vi "Stop.vi"(8 "error in (no error)":errorcluster, 11 "TELEDINE_LECROY in":refnum<class "TELEDINE_LECROY.lvclass">) -> (0 "error out":errorcluster, 3 "TELEDINE_LECROY out":refnum<class "TELEDINE_LECROY.lvclass">)   [LabVIEW 2018, in "TELEDINE_LECROY.lvclass"]
uses:
  TELEDINE_LECROY.lvclass
  C:/Users/Sergey Denisov/Documents/REPS/TRANCON/Classes/GeneralFunctionality/GeneralFunctionality.lvclass
  C:/Users/Sergey Denisov/Documents/REPS/TRANCON/Classes/Oscilloscope/Oscilloscope.lvclass
  GeneralFunctionality/GeneralFunctionality.lvclass/GeneralFunctionality.ctl
  Oscilloscope.lvclass/Oscilloscope.ctl
  LeCroy Wave Series/LeCroy Wave Series.lvlib
  Oscilloscope.lvclass
  GeneralFunctionality/GeneralFunctionality.lvclass
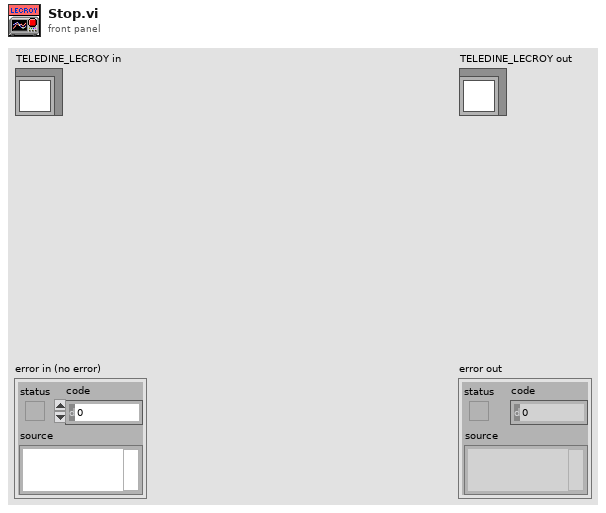
[diagram p1: front panel]
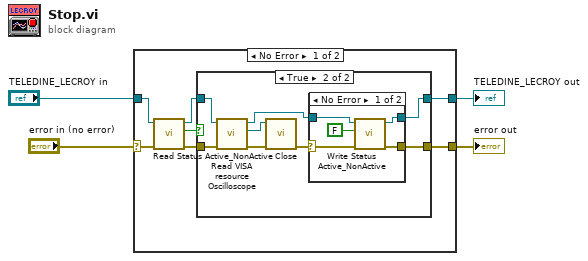
[diagram p0: block diagram]
diagram:
  n1 = case shown="No Error" "error in (no error)" {
    selector: "error in (no error)" -> [w8 w30]
    tunnel: [w11 w30] -> w3
    tunnel: [w10 w29] -> w2
    tunnel: "TELEDINE_LECROY in" -> [w9 w29]
    frame No Error {
      n2 = call "Read Status Active_NonActive.vi"("error in (no error)"=w8, "GeneralFunctionality in"=w9) -> ("error out"=w7:errorcluster, "Status Active/NonActive"=w5:bool, "GeneralFunctionality out"=w6:refnum<class "TELEDINE_LECROY.lvclass">)  [unwired: 7 in]
      n3 = case shown="True" w5 {
        tunnel: w6 -> [w13 w21]
        tunnel: w7 -> [w12 w20]
        tunnel: [w12 w16] -> w11
        tunnel: [w13 w15] -> w10
        frame False {
        }
        frame True {
          n4 = call "Read VISA resource Oscilloscope.vi"("error in (no error)"=w20, "Oscilloscope in"=w21) -> ("error out"=w18:errorcluster, "VISA resource Oscilloscope"=w19:refnum<visa-resource-name>, "Oscilloscope out"=w14:refnum<class "TELEDINE_LECROY.lvclass">)  [unwired: 7 in]
          n5 = call "Close.vi"("error in (no error)"=w18, "VISA resource name"=w19) -> ("error out"=w17:errorcluster)  [unwired: 9 in]
          n6 = case shown="No Error" w17 {
            selector: w17 -> [w25 w27]
            tunnel: [w24 w27] -> w16
            tunnel: [w23 w28] -> w15
            tunnel: w14 -> [w22 w28]
            frame No Error {
              n7 = call "Write Status Active_NonActive.vi"("error in (no error)"=w25, "Status Active/NonActive"=FALSE, "GeneralFunctionality in"=w22) -> ("error out"=w24:errorcluster, "GeneralFunctionality out"=w23:refnum<class "TELEDINE_LECROY.lvclass">)  [unwired: 7 in]
            }
            frame Error {
            }
          }
        }
      }
    }
    frame Error {
    }
  }
  "error out" <- w3
  "TELEDINE_LECROY out" <- w2
